vi "ValidatePathParameter.vi"(8 "error in (no error)":errorcluster, 11 "UI Ref Cluster":T1) -> (0 "error out":errorcluster, 2 "Error Message":string, 3 "UI Ref Cluster Out":T1)   [LabVIEW 2021, in "myRIOMetaDataObj.lvclass"]
uses:
  myRIOMetaDataObj.lvclass
  WizardUIRef.ctl
  AvailableTargets.ctl
  <vilib>/Utility/error.llb/DialogType.ctl
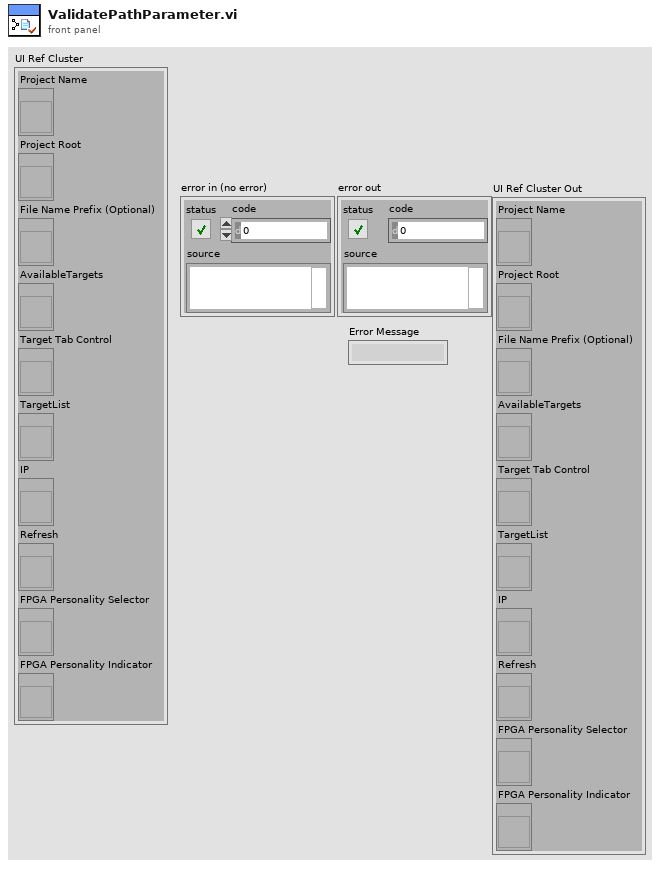
[diagram p1: front panel]
types:
  T1 = typedef "myRIOMetaDataObj.lvclass/WizardUIRef.ctl" = cluster{"Project Name":refnum<vi>, "Project Root":refnum<vi>, "File Name Prefix (Optional)":refnum<vi>, "AvailableTargets":refnum<vi>, "Target Tab Control":refnum<vi>, "TargetList":refnum<vi>, "IP":refnum<vi>, "Refresh":refnum<vi>, "FPGA Personality Selector":refnum<vi>, "FPGA Personality Indicator":refnum<vi>}
  T2 = typedef "DialogType.ctl" = u16
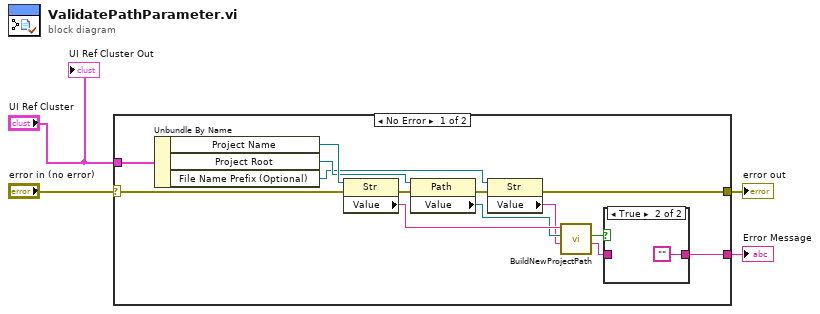
[diagram p0: block diagram]
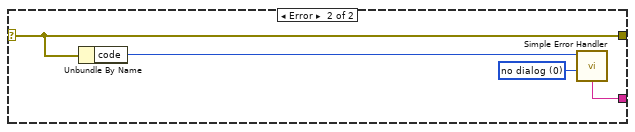
[diagram p3: hidden frame]
diagram:
  n1 = case shown="No Error" "error in (no error)" {
    selector: "error in (no error)" -> [w5 w21]
    tunnel: "UI Ref Cluster" -> [w8 _]
    tunnel: [w7 w22] -> w4
    tunnel: [w6 w21] -> w3
    frame No Error {
      n2 = Unbundle By Name(w8) -> ("Project Name"=w18:refnum<vi>, "Project Root"=w16:refnum<vi>, "File Name Prefix (Optional)"=w13:refnum<vi>)
      n3 = property class="Str"(reference=w18, error in=w5) -> (error out=w17:errorcluster, "Value"=w15:string)  [unwired: 1 out]
      n4 = property class="Path"(reference=w16, error in=w17) -> (error out=w12:errorcluster, "Value"=w14:path)  [unwired: 1 out]
      n5 = property class="Str"(reference=w13, error in=w12) -> (error out=w6:errorcluster, "Value"=w11:string)  [unwired: 1 out]
      n6 = call <resource>:"BuildNewProjectPath.vi"("File Prefix"=w11, "Project Root"=w14, "Project Name"=w15) -> ("Error Message"=w9:string, "Valid?"=w10:bool)  [unwired: 6 in, 1 out]
      n7 = case shown="True" w10 {
        tunnel: w9 -> [w19 _]
        tunnel: [w19 ""] -> w7
        frame False {
        }
        frame True {
        }
      }
    }
    frame Error {
      w23 = T2 0 items=["no dialog", "OK message", "continue or stop message", "OK message + warnings", "continue/stop + warnings"] ("type of dialog (OK msg:1)")
      n8 = Unbundle By Name(w21) -> ("code"=w24:i32)
      n9 = call <vilib>:"Simple Error Handler.vi"("error code (no error:0)"=w24, "type of dialog (OK msg:1)"=w23) -> ("message"=w22:string)  [unwired: 3 in, 4 out]
    }
  }
  "Error Message" <- w4
  "error out" <- w3
  "UI Ref Cluster Out" <- "UI Ref Cluster"
